vi "sv_Insert Swept Scaled Response Magnitude.vi"(4 "AI index":i32, 6 "read/write indices":T1(array[cluster]), 9 "unscaled response magnitude":dbl format="%.2f", 10 "AI freq index":i32, 11 "measurements in":T2 {"scaled response magnitude" format="%.3f"; "Harm[]" format="%.2f"; "THD" format="%.2f"; "Im [response]" format="%.2f"; "Re [response]" format="%.2f"; "Im [stimulus]" format="%.2f"; "Re [stimulus]" format="%.2f"; "RMS response" format="%.2f"; "RMS stimulus" format="%.2f"}) -> (3 "measurements out":T2 {"scaled response magnitude" format="%.3f"; "Harm[]" format="%.2f"; "THD" format="%.2f"; "Im [response]" format="%.2f"; "Re [response]" format="%.2f"; "Im [stimulus]" format="%.2f"; "Re [stimulus]" format="%.2f"; "RMS response" format="%.2f"; "RMS stimulus" format="%.2f"})   [LabVIEW 2017, in "SoundVib_SweptSine.lvlib"]
uses:
  <vilib>/addons/Sound and Vibration/svt_Swept Sine/SoundVib_SweptSine.lvlib
  <vilib>/addons/Sound and Vibration/svt_Swept Sine/subVIs/sv_Swept Sine Measurements.ctl
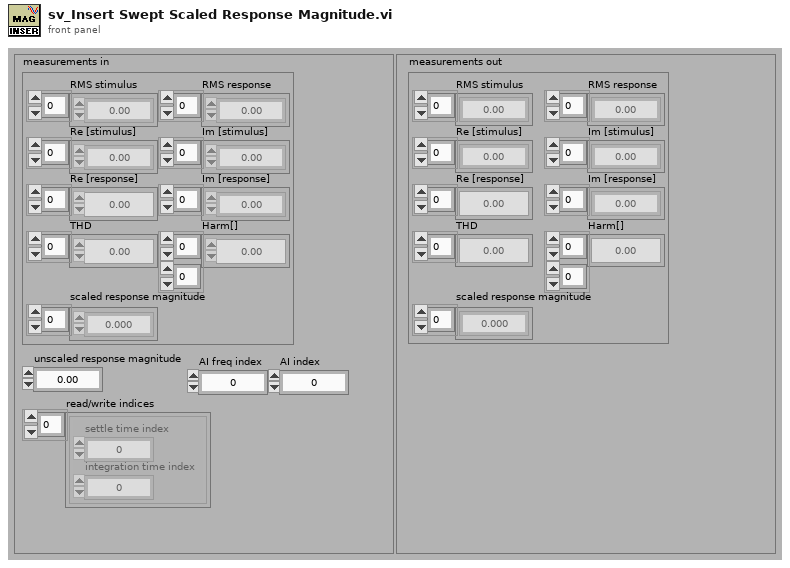
[diagram p1: front panel]
types:
  T1 = cluster{"settle time index":u32, "integration time index":u32}[]
  T2 = typedef "SoundVib_SweptSine.lvlib/sv_Swept Sine Measurements.ctl" = cluster{"RMS stimulus":dbl[], "RMS response":dbl[], "Re [stimulus]":dbl[], "Im [stimulus]":dbl[], "Re [response]":dbl[], "Im [response]":dbl[], "THD":dbl[], "Harm[]":dbl[][], "scaled response magnitude":dbl[]}
  T3 = cluster{"settle time index":u32, "integration time index":u32}
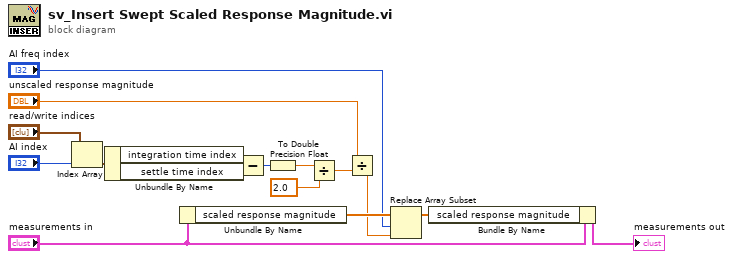
[diagram p0: block diagram]
diagram:
  n1 = Index Array(array="read/write indices", index="AI index") -> (element=w11:T3)
  n2 = Unbundle By Name(w11) -> ("integration time index"=w10:u32, "settle time index"=w9:u32)
  n3 = Unbundle By Name("measurements in") -> ("scaled response magnitude"=w12:dbl[])
  n4 = Subtract(x=w10, y=w9) -> (x-y=w3:u32)
  n5 = To Double Precision Float(number=w3) -> (double precision float=w1:dbl)
  n6 = Divide(x=w1, y=2.0) -> (x/y=w2:dbl)
  n7 = Divide(x="unscaled response magnitude", y=w2) -> (x/y=w8:dbl)
  n8 = Replace Array Subset(array=w12, new element=w8, index="AI freq index") -> (w13:dbl[])
  n9 = Bundle By Name(cluster="measurements in", "scaled response magnitude"=w13) -> (→"measurements out":T2)
